vi "Open from SFTP.vi"(4 "Permissions":T2={"Owner"={"Read"=TRUE, "Write"=TRUE, "Execute"=FALSE}, "Group"={"Read"=TRUE, "Write"=FALSE, "Execute"=FALSE}, "Others"={"Read"=TRUE, "Write"=FALSE, "Execute"=FALSE}}, 6 "Options":T1={"Read"=TRUE, "Write"=TRUE, "Append"=FALSE, "Create"=FALSE, "Truncate"=FALSE, "Exclude"=FALSE}, 8 "Error In":errorcluster, 10 "Remote Path":string, 11 "SFTP":refnum<class "SFTP.lvclass">) -> (0 "Error Out":errorcluster, 3 "SFTP File":refnum<class "SFTP File.lvclass">)   [LabVIEW 2021, in "Field_RnD_Services_LIBSSH2_Toolkit.lvlib" / "SFTP File.lvclass"]
doc: "Creates a new SFTP File object from a SFTP object."
uses:
  220524-VNA RP FLAT.llb/SFTP File.lvclass
  220524-VNA RP FLAT.llb/SFTP.lvclass
  220524-VNA RP FLAT.llb/Permissions.ctl
  Field_RnD_Services_LIBSSH2_Toolkit/Modes.ctl
  220524-VNA RP FLAT.llb/Open Options.ctl
  220524-VNA RP FLAT.llb/SFTP File.lvclass/SFTP File.ctl
  220524-VNA RP FLAT.llb/Field_RnD_Services_LIBSSH2_Toolkit.lvlib
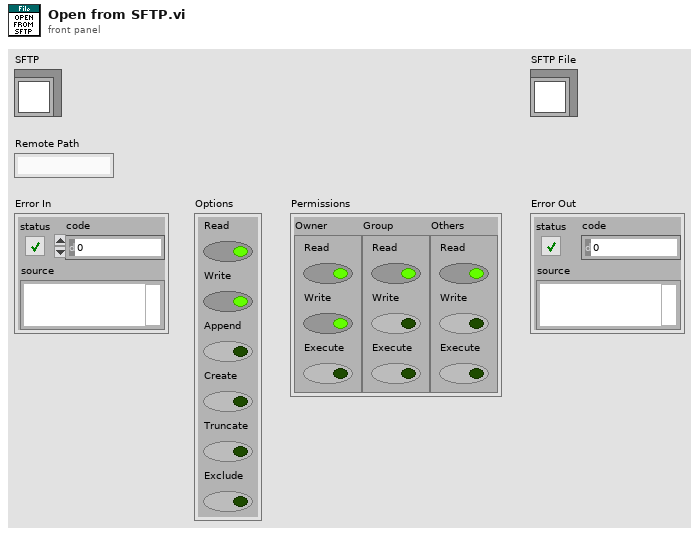
[diagram p1: front panel]
types:
  T1 = typedef "Field_RnD_Services_LIBSSH2_Toolkit.lvlib/SFTP File.lvclass/Open Options.ctl" = cluster{"Read":bool, "Write":bool, "Append":bool, "Create":bool, "Truncate":bool, "Exclude":bool}
  T2 = typedef "Field_RnD_Services_LIBSSH2_Toolkit.lvlib/Permissions.ctl" = cluster{"Owner":T3, "Group":T3, "Others":T3}
  T3 = typedef "Field_RnD_Services_LIBSSH2_Toolkit.lvlib/Modes.ctl" = cluster{"Read":bool, "Write":bool, "Execute":bool}
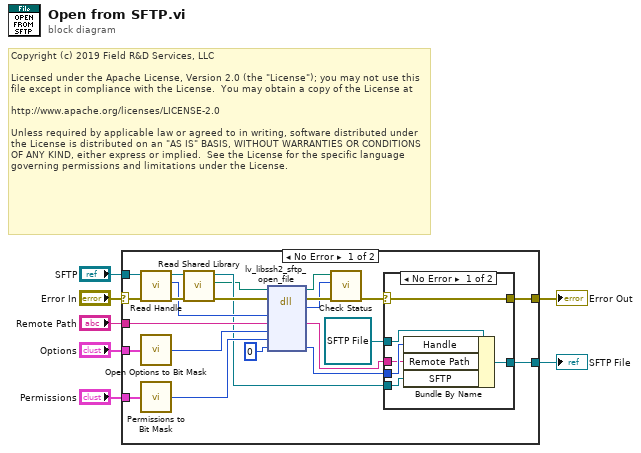
[diagram p0: block diagram]
diagram:
  # "Copyright (c) 2019 Field R&D Services, LLC\n\nLicensed under the Apache License, Version 2.0 (the \"License\"); you may not use this file except in compliance with the License.  You may obtain a copy of the License at\n\nhttp://www.apache.org/licenses/LICENSE-2.0\n\nUnless required by applicable law or agreed to in writing, software distributed under the License is distributed on an \"AS IS\" BASIS, WITHOUT WARRANTIES OR CONDITIONS OF ANY KIND, either express or implied.  See the License for the specific language governing permissions and limitations under the License."
  n1 = case shown="No Error" "Error In" {
    selector: "Error In" -> [w24 w39]
    tunnel: [w9 w39] -> w6
    tunnel: "SFTP" -> [w25 _]
    tunnel: "Remote Path" -> [w30 _]
    tunnel: [w17 _] -> w3
    tunnel: "Permissions" -> [w16 _]
    tunnel: "Options" -> [w14 _]
    frame No Error {
      n2 = call "Read Handle.vi"("Error In"=w24, "SFTP In"=w25) -> ("Erorr Out"=w22:errorcluster, "Handle"=w21:u64, "SFTP Out"=w23:refnum<class "SFTP.lvclass">)  [unwired: 7 in]
      n3 = call "Open Options to Bit Mask.vi"("Options"=w14) -> ("Bit Mask"=w13:u32)
      n4 = call "Permissions to Bit Mask.vi"("Permissions"=w16) -> ("Bit Mask"=w15:u32)
      n5 = call "Read Shared Library.vi"("Error In"=w22, "SFTP In"=w23) -> ("Erorr Out"=w20:errorcluster, "libssh2lv Shared Library"=w11:path, "SFTP Out"=w12:refnum<class "SFTP.lvclass">)  [unwired: 7 in]
      n6 = dll-call lib="D:/Users/cfield/Code/Field R&D Services/SSH/LV-LIBSSH2/LabVIEW/trunk/src/Toolkit/Support/lv-libssh2.*" fn="lv_libssh2_sftp_open_file"(path in=w11, error in=w20, "sftp"=w21, "path"=w30, "flags"=w13, "permissions"=w15, "handle"=u64 0) -> (path out=w29:path, error out=w28:errorcluster, "status"=w27:i32, "path"=w8:string, "handle"=w18:u64)  [unwired: 4 in]
      n7 = call "Check Status.vi"("Error In"=w28, "Status"=w27, "libssh2lv Shared Library In"=w29) -> ("Error Out"=w10:errorcluster)  [unwired: 7 in, 1 out]
      n8 = case shown="No Error" w10 {
        selector: w10 -> [w32 w37]
        tunnel: refnum<class "SFTP File.lvclass"> refnum ("Toolkit.lvlib:SFTP File.lvclass") -> [w36 w38]
        tunnel: w18 -> [w35 _]
        tunnel: [w34 w38] -> w17
        tunnel: w12 -> [w33 _]
        tunnel: [w32 w37] -> w9
        tunnel: w8 -> [w31 _]
        frame No Error {
          n9 = Bundle By Name(cluster=w36, "Handle"=w35, "Remote Path"=w31, "SFTP"=w33) -> (w34:refnum<class "SFTP File.lvclass">)
        }
        frame Error {
        }
      }
    }
    frame Error {
    }
  }
  "Error Out" <- w6
  "SFTP File" <- w3
